vi "StateN.vi"(0 "Start":bool, 1 "Stop":bool, 2 "Reset":bool, 3 "T_table":u32[][](array[numeric])=[[3000, 1, 2, 2], [3000, 2, 3, 3], [3000, 3, 4, 4], [3000, 0, 0, 0]], 4 "C_table":cluster{"C":bool, "NC":u32}[][](array[cluster]), 7 "End step":u32=4) -> (11 "N next":u32, 14 "Start":bool, 15 "Stop":bool, 16 "End":bool, 17 "t":u32, 18 "N curr":u32)   [LabVIEW 2019, in "Userlib.lvlib"]
uses:
  Userlib.lvlib
  Trigers/Triggers.lvlib
  Timer Delay/Timers.lvlib
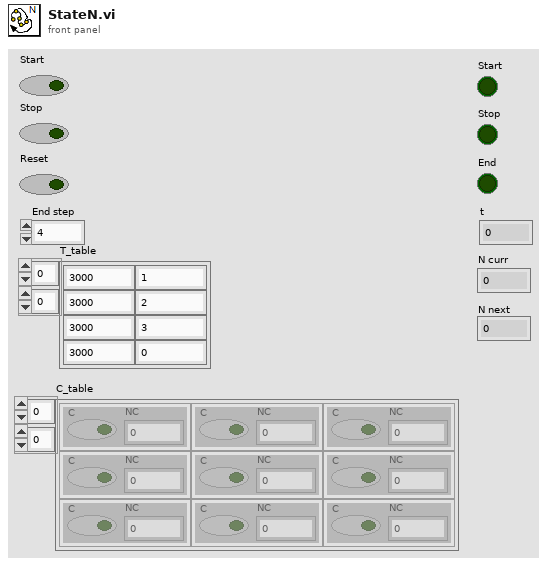
[diagram p1: front panel]
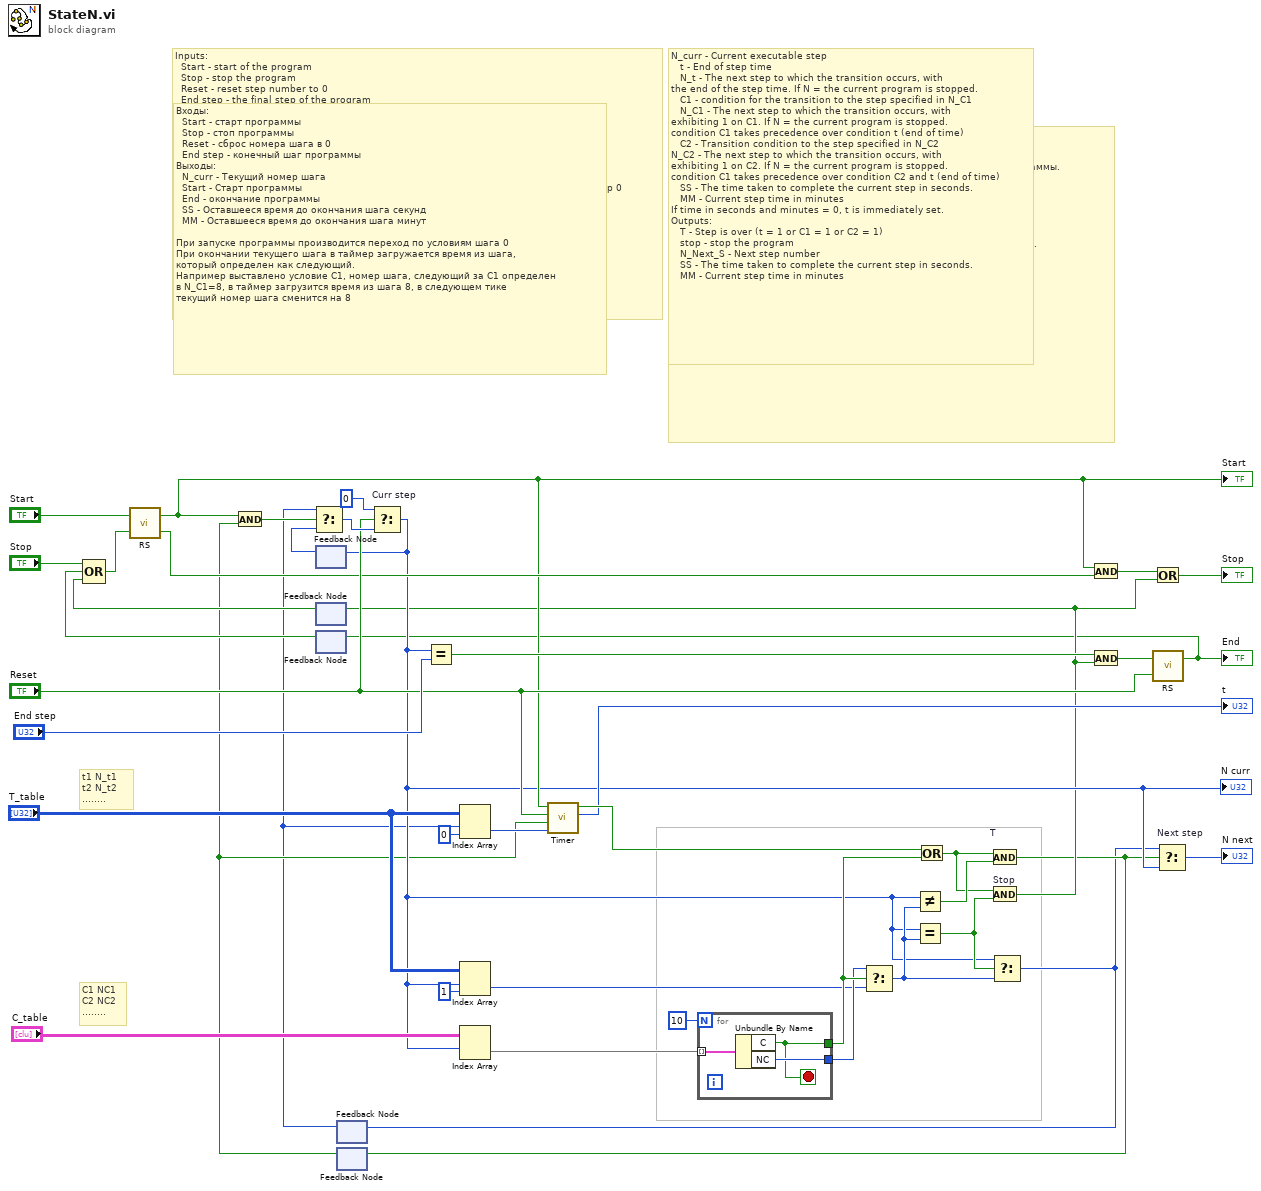
[diagram p0: block diagram]
diagram:
  # "C1 NC1\nC2 NC2\n........"
  # "t1 N_t1\nt2 N_t2\n........"
  # "N_curr - Current executable step\n   t - End of step time\n   N_t - The next step to which the transition occurs, with\nthe end of the step time. If N = the current program is stopped.\n   C1 - condition for the transition to the step specified in N_C1\n   N_C1 - The next step to which the transition occurs, with\nexhibiting 1 on C1. If N = the current program is stopped.\ncondition C1 takes precedence over condition t (end of time)\n   C2 - Transition condition to the step specified in N_C2\nN_C2 - The next step to which the transition occurs, with\nexhibiting 1 on C2. If N = the current program is stopped.\ncondition C1 takes precedence over condition C2 and t (end of time)\n   SS - The time taken to complete the current step in seconds.\n   MM - Current step time in minutes\nIf time in seconds and minutes = 0, t is immediately set.\nOutputs:\n   T - Step is over (t = 1 or C1 = 1 or C2 = 1)\n   stop - stop the program\n   N_Next_S - Next step number\n   SS - The time taken to complete the current step in seconds.\n   MM - Current step time in minutes"
  # "Inputs:\n  Start - start of the program\n  Stop - stop the program\n  Reset - reset step number to 0\n  End step - the final step of the program\nOutputs:\n  N_curr - Current step number\n  Start - Start of the program\n  End - the end of the program\n  SS - Time remaining until the end of the step seconds\n  MM - Time remaining until the end of the step minutes\n\nWhen starting the program, the transition is performed according to the conditions of step 0\nAt the end of the current step, the time from the step is loaded into the timer,\nwhich is defined as the following.\nFor example, condition C1 is set, the step number following C1 is defined\nin N_C1 = 8, the time from step 8 is loaded into the timer, in the next tick\nthe current step number will change to 8"
  # "N_curr - Текущий выполняемый шаг\n  t - Окончание времени шага\n  N_t - Следующий шаг, к которому происходит переход, при\nокончании времени шага. Если N = текущему происходит останов программы.\n  C1 - Условие перехода к шагу, указанному в N_C1\n  N_C1 - Следующий шаг, к которому происходит переход, при\nвыставлении 1 на С1. Если N =текущему происходит останов программы.\nусловие С1 имеет приоритет над условием t (окончание времени)\n  C2 - Условие перехода к шагу, указанному в N_C2\n  N_C2 - Следующий шаг, к которому происходит переход, при\nвыставлении 1 на С2. Если N = текущему происходит останов программы.\nусловие С1 имеет приоритет над условием С2 и t (окончание времени)\n  SS - Время выполнения текущего шага в секундах\n  MM - Время выполнения текущего шага в минутах\nЕсли время в секундах и минутах = 0, сразу выставляется t\nВыходы:\n  T - Шаг окончен (t=1 или C1=1 или С2=1)\n  stop - остановить программу\n  N_Next_S - Номер следующего шага\n  SS - Время выполнения текущего шага в секундах\n  MM - Время выполнения текущего шага в минутах"
  # "Входы:\n  Start - старт программы\n  Stop - стоп программы\n  Reset - сброс номера шага в 0\n  End step - конечный шаг программы\nВыходы:\n  N_curr - Текущий номер шага\n  Start - Старт программы\n  End - окончание программы\n  SS - Оставшееся время до окончания шага секунд\n  MM - Оставшееся время до окончания шага минут\n\nПри запуске программы производится переход по условиям шага 0\nПри окончании текущего шага в таймер загружается время из шага,\nкоторый определен как следующий.\nНапример выставлено условие C1, номер шага, следующий за С1 определен\nв N_C1=8, в таймер загрузится время из шага 8, в следующем тике \nтекущий номер шага сменится на 8"
  n1 = feedback #1() -> (w9:u32)  [unwired: 1 in]
  n2 = feedback #2() -> (w7:bool)  [unwired: 1 in]
  n3 = feedback #3() -> (w5:bool)  [unwired: 1 in]
  n4 = Compound Arithmetic op=OR("Stop", w5, w7) -> (w40:bool)
  n5 = call "RS.vi"("R"=w40, "S"="Start") -> ("~Q"=w25:bool, "Q"=w11:bool)
  "Start" <- w11
  n6 = feedback #4() -> (w1:u32)  [unwired: 1 in]
  n7 = feedback #5() -> (w3:bool)  [unwired: 1 in]
  n8 = And(x=w11, y=w3) -> (x .and. y?=w41:bool)
  n9 = Select(t=w1, s=w41, f=w9) -> (s? t:f=w31:u32)
  n10 = Select "Curr step"(t=u32 0, s="Reset", f=w31) -> (s? t:f=w10:u32)
  "N curr" <- w10
  n11 = feedback-in #1(w10) -> ()
  n12 = Equal?(x=w10, y="End step") -> (x = y?=w28:bool)
  n13 = Index Array(array="T_table", index (row)=w1, index (col)=0 ("disabled index (col)")) -> (element=w13:u32)
  n14 = Index Array(array="T_table", index (row)=w10, index (col)=1 ("disabled index (col)")) -> (element=w15:u32)
  n15 = Index Array(array="C_table", index (row)=w10) -> (element=w12:cluster{"C":bool, "NC":u32}[])  [unwired: 1 in]
  n16 = call "Timer.vi"("ms"=w13, "Load (F)"=w3, "Reset (F)"="Reset", "Start (T)"=w11) -> ("t ms"=→"t":u32, "End"=w32:bool)  [unwired: 5 in]
  n17 = for {
    N: 10 -> [_]
    tunnel: w12 -> [w44] mode=indexing
    tunnel: [w43] -> w19
    tunnel: [w42] -> w20
    stop <- w42 stop-if-true
    n18 = Unbundle By Name(w44) -> ("C"=w42:bool, "NC"=w43:u32)
  }
  n19 = Select(t=w19, s=w20, f=w15) -> (s? t:f=w24:u32)
  n20 = Not Equal?(x=w10, y=w24) -> (x != y?=w35:bool)
  n21 = Equal?(x=w10, y=w24) -> (x = y?=w33:bool)
  n22 = Or(x=w32, y=w20) -> (x .or. y?=w34:bool)
  n23 = And "T"(x=w34, y=w35) -> (x .and. y?=w4:bool)
  n24 = feedback-in #5(w4) -> ()
  n25 = And "Stop"(x=w34, y=w33) -> (x .and. y?=w8:bool)
  n26 = feedback-in #2(w8) -> ()
  n27 = Select(t=w10, s=w33, f=w24) -> (s? t:f=w2:u32)
  n28 = feedback-in #4(w2) -> ()
  n29 = And(x=w11, y=w25) -> (x .and. y?=w27:bool)
  n30 = And(x=w28, y=w8) -> (x .and. y?=w37:bool)
  n31 = Or(x=w27, y=w8) -> (x .or. y?=→"Stop":bool)
  n32 = call "RS.vi"("R"="Reset", "S"=w37) -> ("Q"=w6:bool)  [unwired: 1 out]
  "End" <- w6
  n33 = feedback-in #3(w6) -> ()
  n34 = Select "Next step"(t=w2, s=w4, f=w10) -> (s? t:f=→"N next":u32)
